vi "Test.vi"   [LabVIEW 2015, in "Sequencer.lvclass"]
uses:
  Sequencer.lvclass
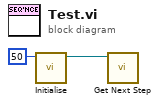
[diagram p0: block diagram]
diagram:
  n1 = call "Initialise.vi"("Max Steps (100)"=50) -> ("Sequencer out"=w1:refnum<class "Sequencer.lvclass">)  [unwired: 9 in, 1 out]
  n2 = call "Get Next Step.vi"("Sequencer in"=w1) -> ()  [unwired: 6 in, 5 out]
